vi "COMI Load Device.vi"(10 "instance":u32, 11 "deviceID":u16) -> (3 "function return":u32)   [LabVIEW 2017, in "Comidll.lvlib"]
doc: "HANDLE (COMI_LoadDevice) (unsigned short deviceID, unsigned long instance);"
uses:
  <userlib>/Comidll/Comidll.lvlib
  <userlib>/Comidll/Comidll.dll
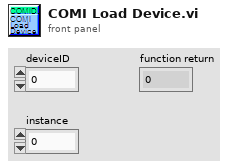
[diagram p1: front panel]
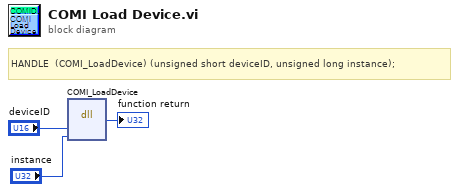
[diagram p0: block diagram]
diagram:
  # "HANDLE \t(COMI_LoadDevice) (unsigned short deviceID, unsigned long instance);"
  n1 = dll-call lib="C:/Program Files/National Instruments/LabVIEW 2017/user.lib/Comidll/Comidll.*" fn="COMI_LoadDevice"("deviceID"="deviceID", "instance"="instance") -> (→"function return":u32)  [unwired: 5 in, 2 out]
